vi "Drive Forward.vi"(8 "error in (no error)":errorcluster, 9 "Distance":dbl, 10 "rightDistance":T1={"DevStatus"={"status"=FALSE, "code"=0, "source"=""}, "EncoderIndex"=enum."Invalid", "CounterIndex"=enum."Ctr 1", "DistancePerCount"=2.0, "Decoding Type"=enum."4x"}, 11 "leftDistance":T1={"DevStatus"={"status"=FALSE, "code"=0, "source"=""}, "EncoderIndex"=enum."Invalid", "CounterIndex"=enum."Ctr 1", "DistancePerCount"=2.0, "Decoding Type"=enum."4x"}) -> (0 "error out":errorcluster, 2 "rightDistance":T1, 3 "leftDistance":T1, 4 "Stop":bool)   [LabVIEW 2017]
uses:
  <vilib>/Rock Robotics/WPI/Encoder/WPI_EncoderDevRef.ctl
  <vilib>/Rock Robotics/SystemInterfaces/Encoder/FPGA_EncoderIdx.ctl
  <vilib>/Rock Robotics/SystemInterfaces/Counter/FPGA_CounterCtrSystemIndex.ctl
  <vilib>/Rock Robotics/WPI/Encoder/WPI_EncoderType.ctl
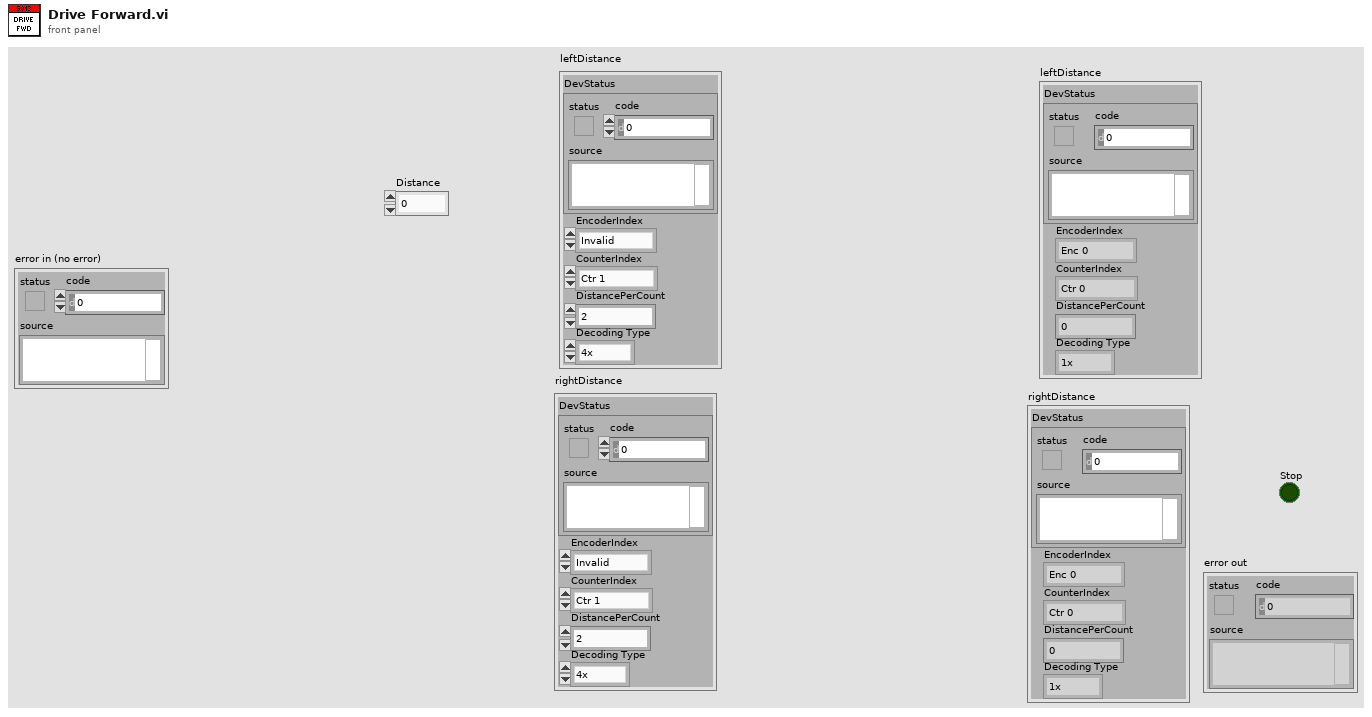
[diagram p1: front panel]
types:
  T1 = typedef "WPI_EncoderDevRef.ctl" = cluster{"DevStatus":errorcluster, "EncoderIndex":T2, "CounterIndex":T3, "DistancePerCount":dbl, "Decoding Type":T4}
  T2 = typedef "FPGA_EncoderIdx.ctl" = enum8{"Enc 0", "Enc 1", "Enc 2", "Enc 3", "Enc 4", "Enc 5", "Enc 6", "Enc 7", "Invalid"}
  T3 = typedef "FPGA_CounterCtrSystemIndex.ctl" = enum8{"Ctr 0", "Ctr 1", "Ctr 2", "Ctr 3", "Ctr 4", "Ctr 5", "Ctr 6", "Ctr 7", "Invalid"}
  T4 = typedef "WPI_EncoderType.ctl" = enum16{"1x", "2x", "4x"}
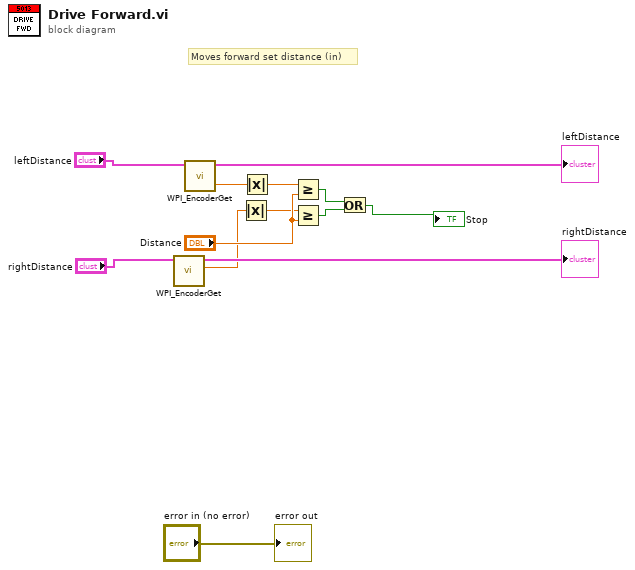
[diagram p0: block diagram]
diagram:
  # "Moves forward set distance (in)"
  n1 = call <vilib>:"WPI_EncoderGet.vi"("EncoderDevRef"="rightDistance") -> ("Distance"=w7:dbl, "EncoderDevRef"=→"rightDistance":T1)  [unwired: 5 in, 4 out]
  n2 = call <vilib>:"WPI_EncoderGet.vi"("EncoderDevRef"="leftDistance") -> ("Distance"=w8:dbl, "EncoderDevRef"=→"leftDistance":T1)  [unwired: 5 in, 4 out]
  n3 = Absolute Value(x=w7) -> (abs(x)=w3:dbl)
  n4 = Absolute Value(x=w8) -> (abs(x)=w4:dbl)
  n5 = Greater Or Equal?(x=w4, y="Distance") -> (x >= y?=w6:bool)
  n6 = Greater Or Equal?(x=w3, y="Distance") -> (x >= y?=w5:bool)
  n7 = Or(x=w6, y=w5) -> (x .or. y?=→"Stop":bool)
  "error out" <- "error in (no error)"
